vi "close.vi"(8 "error in (no error)":errorcluster, 11 "Thermocouples in":refnum<class "Thermocouples.lvclass">) -> (0 "error out":errorcluster, 3 "Thermocouples out":refnum<class "Thermocouples.lvclass">)   [LabVIEW 2025, in "Thermocouples.lvclass"]
uses:
  Thermocouples.lvclass
  Thermocouples.lvclass/Thermocouples.ctl
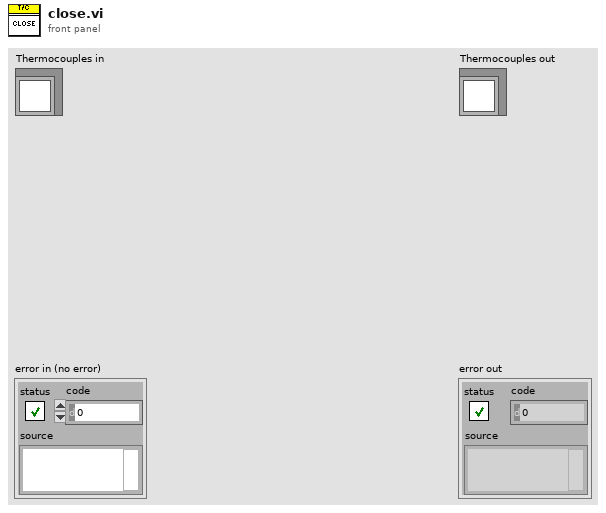
[diagram p1: front panel]
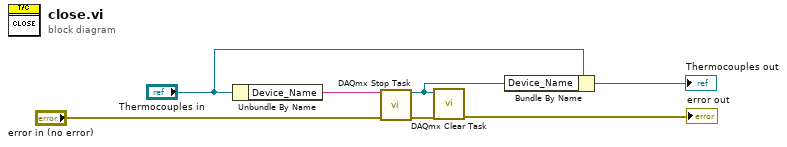
[diagram p0: block diagram]
diagram:
  n1 = Unbundle By Name("Thermocouples in") -> ("Device_Name"=w3:string)
  n2 = call <vilib>:"DAQmx Stop Task.vi"("task/channels in"=w3, "error in"="error in (no error)") -> ("task out"=w1:refnum<k21>, "error out"=w6:errorcluster)  [unwired: 12 in]
  n3 = call <vilib>:"DAQmx Clear Task.vi"("task in"=w1, "error in"=w6) -> ("error out"=→"error out":errorcluster)  [unwired: 13 in]
  n4 = Bundle By Name(cluster="Thermocouples in", "Device_Name"=w1) -> (→"Thermocouples out":refnum<class "Thermocouples.lvclass">)
